vi "RSNRPZ Get Scope Averaging State.vi"(8 "error in (no error)":errorcluster, 10 "Channel (1)":i32=1, 11 "VISA session":refnum<visa-resource-name> caption="VISA resource name") -> (0 "error out":errorcluster, 2 "Scope Averaging":bool, 3 "dup VISA session":refnum<visa-resource-name> caption="VISA resource name")   [LabVIEW 2010]
doc: "This VI reads the state of filter function of a sensor.\n\nNote:\n\n1) This VI is not available for NRP-Z51.\n\nRemote-control command(s):\nSENS:TRAC:AVER:STAT?"
uses:
  rsnrpz_32.dll
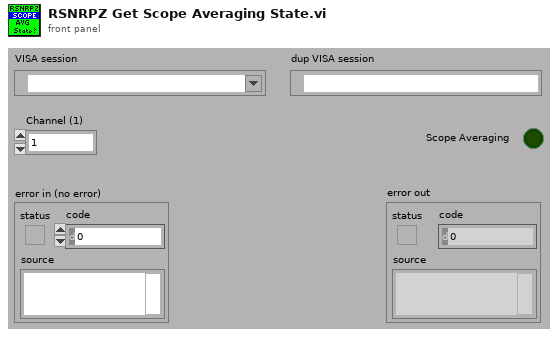
[diagram p1: front panel]
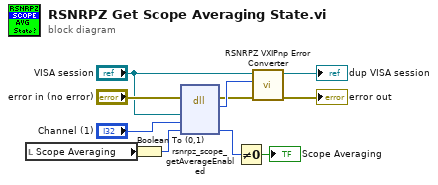
[diagram p0: block diagram]
diagram:
  n1 = local read "Scope Averaging"() -> (w9:bool)
  n2 = Boolean To (0,1)(Boolean=w9) -> (0, 1=w7:i16)
  n3 = dll-call lib="rsnrpz_32.dll" fn="rsnrpz_scope_getAverageEnabled"(error in="error in (no error)", "VISA Session"="VISA session", "Channel"="Channel (1)", "Scope Averaging"=w7) -> (error out=w5:errorcluster, "Status"=w11:i32, "Scope Averaging"=w8:u16)  [unwired: 4 in, 1 out]
  n4 = Not Equal To 0?(x=w8) -> (x != 0?=→"Scope Averaging":bool)
  n5 = call <instrlib>:"RSNRPZ VXIPnp Error Converter.vi"("error in"=w5, "VXIPnp error code"=w11, "VISA session"="VISA session") -> ("error out"=→"error out":errorcluster, "dup VISA session"=→"dup VISA session":refnum<visa-resource-name>)  [unwired: 7 in]
